vi "Main.vi"() -> ()   [LabVIEW 2019]
uses:
  <vilib>/DAQmx/miscellaneous.llb/DAQmx Fill In Error Info.vi
  <vilib>/DAQmx/create/channels.llb/DAQmx Create Channel (AI-Temperature-Thermocouple).vi
  <vilib>/DAQmx/configure/timing.llb/DAQmx Timing (Sample Clock).vi
  <vilib>/DAQmx/read.llb/DAQmx Read (Analog DBL 1Chan 1Samp).vi
  <resource>/objmgr/daqmx.rc
panel:
  out "Threshold Exceeded?":bool
  in  "Temperature threshold (deg C)":dbl=100.0
  out "Waveform Chart":dbl(graph)
  out "Actual Sample Rate (Hz)":dbl=1.0 format="%#_13g"
  in  "Number of Samples":i32=100
  in  "Desired Sample Rate (Hz)":dbl=1000.0 format="%#_13g"
  in  "Thermocouple Channel":tag="PCI-6221/ai0"
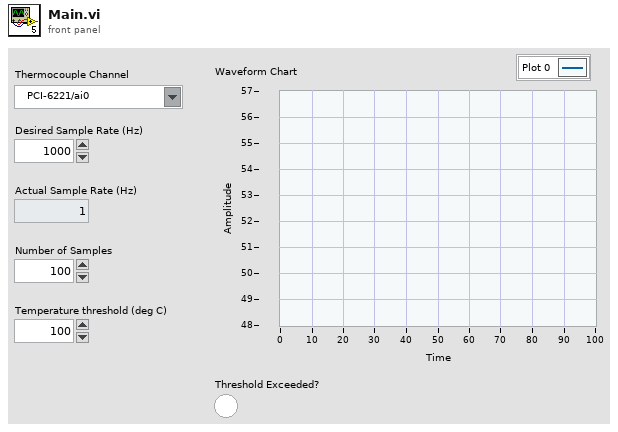
[diagram p1: front panel]
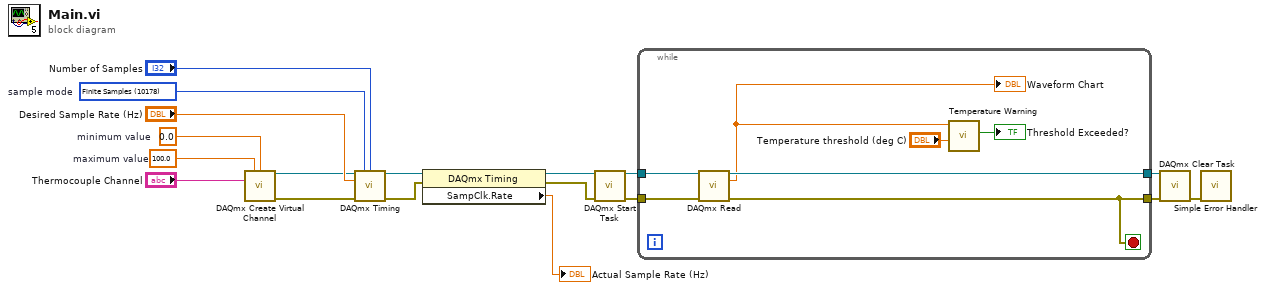
[diagram p0: block diagram]
diagram:
  w12 = 100.0  # maximum value
  w13 = 0.0  # minimum value
  w18 = 10178 items=["Finite Samples"=10178, "Continuous Samples"=10123, "Hardware Timed Single Point"=12522]  # sample mode
  n1 = call-poly <vilib>:"DAQmx Create Virtual Channel.vi"("maximum value"=w12, "minimum value"=w13, "physical channels"="Thermocouple Channel") -> ("task out"=w16:refnum<k21>, "error out"=w15:errorcluster)  [unwired: 11 in]
  n2 = call-poly <vilib>:"DAQmx Timing.vi"("task/channels in"=w16, "sample mode"=w18, "samples per channel"="Number of Samples", "rate"="Desired Sample Rate (Hz)", "error in"=w15) -> ("task out"=w10:refnum<k21>, "error out"=w9:errorcluster)  [unwired: 9 in]
  n3 = property class="DAQmx Timing"(reference=w10, error in=w9) -> (reference out=w8:refnum<k21>, error out=w7:errorcluster, "SampClk.Rate"=→"Actual Sample Rate (Hz)":dbl)
  n4 = call <vilib>:"DAQmx Start Task.vi"("task/channels in"=w8, "error in"=w7) -> ("task out"=w5:refnum<k21>, "error out"=w4:errorcluster)  [unwired: 12 in]
  n5 = while {
    tunnel: w5 -> [w25]
    tunnel: [w23] -> w3
    tunnel: w4 -> [w24]
    tunnel: [w19] -> w2
    stop <- w19 stop-if-true
    n6 = call-poly <vilib>:"DAQmx Read.vi"("task/channels in"=w25, "error in"=w24) -> ("task out"=w23:refnum<k21>, "data"=w21:dbl, "error out"=w19:errorcluster)  [unwired: 11 in]
    "Waveform Chart" <- w21
    n7 = call "Temperature Warning.vi"("Threshold"="Temperature threshold (deg C)", "Current Temperature"=w21) -> ("Threshold Exceeded?"=→"Threshold Exceeded?":bool)  [unwired: 9 in]
  }
  n8 = call <vilib>:"DAQmx Clear Task.vi"("task in"=w3, "error in"=w2) -> ("error out"=w1:errorcluster)  [unwired: 13 in]
  n9 = call <vilib>:"Simple Error Handler.vi"("error in (no error)"=w1) -> ()  [unwired: 4 in, 5 out]
